vi "Methode 1.vi"(8 "error in (no error)":errorcluster, 11 "ID in":refnum<class "ID.lvclass">) -> (0 "error out":errorcluster, 3 "ID out":refnum<class "ID.lvclass">)   [LabVIEW 2023, in "ID.lvclass"]
uses:
  ID.lvclass
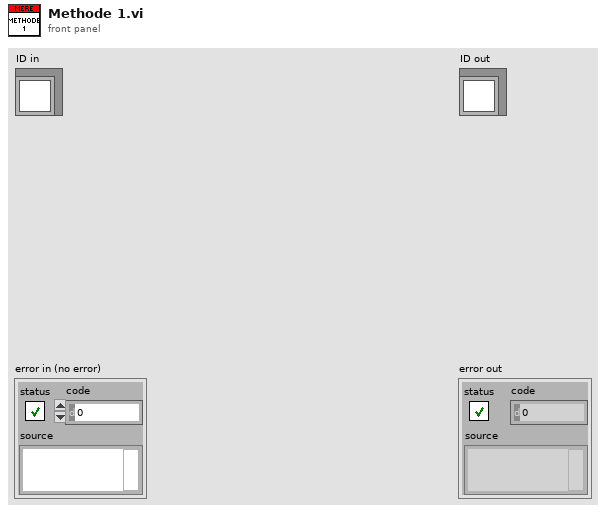
[diagram p1: front panel]
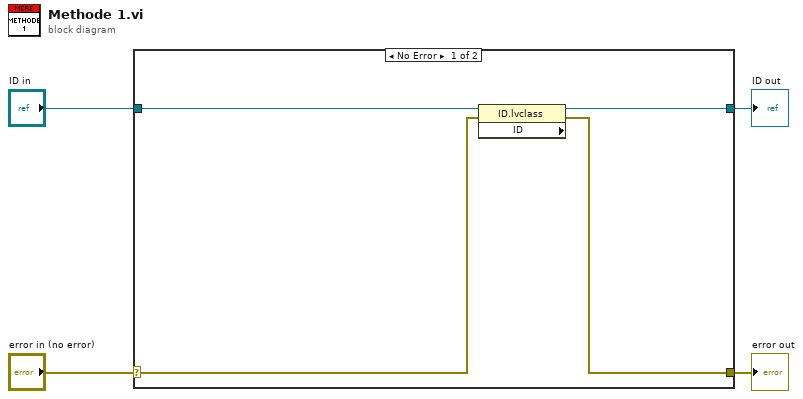
[diagram p0: block diagram]
diagram:
  n1 = case shown="No Error" "error in (no error)" {
    selector: "error in (no error)" -> [w7 w10]
    tunnel: [w6 w10] -> w3
    tunnel: [w5 w9] -> w1
    tunnel: "ID in" -> [w8 w9]
    frame No Error {
      n2 = property class="ID.lvclass" props=["ID"](reference=w8, error in=w7) -> (reference out=w5:refnum<class "ID.lvclass">, error out=w6:errorcluster)  [unwired: 1 out]
    }
    frame Error {
    }
  }
  "error out" <- w3
  "ID out" <- w1
